vi "空载计算.vi"(10 "扭矩数组":dbl[](array[numeric])) -> (0 "空载扭差":dbl format="%#.2f", 1 "空载平均扭矩":dbl format="%#.2f", 2 "空载最小扭矩":dbl, 3 "空载峰值扭矩":dbl format="%#.2f")   [LabVIEW 2011]
panel:
  out "第一个子数组":dbl[](array[numeric])
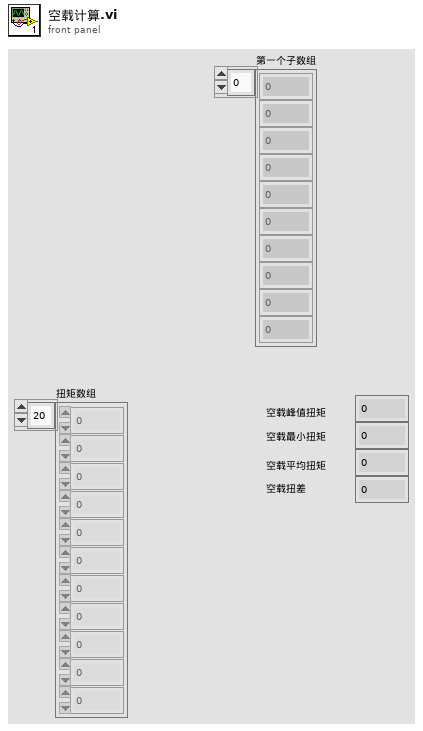
[diagram p1: front panel]
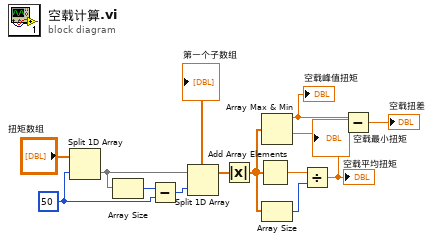
[diagram p0: block diagram]
diagram:
  w3 = 50 ("索引")
  n1 = Split 1D Array(array="扭矩数组", index=w3) -> (second subarray=w5:dbl[])  [unwired: 1 out]
  n2 = Array Size(array=w5) -> (size(s)=w4:i32)
  n3 = Subtract(x=w4, y=w3) -> (x-y=w2:i32)
  n4 = Split 1D Array(array=w5, index=w2) -> (first subarray=w9:dbl[])  [unwired: 1 out]
  "第一个子数组" <- w9
  n5 = Absolute Value(x=w9) -> (abs(x)=w11:dbl[])
  n6 = Add Array Elements(numeric array=w11) -> (sum=w12:dbl)
  n7 = Array Max & Min(array=w11) -> (max value=w8:dbl, min value=→"空载最小扭矩":dbl)  [unwired: 2 out]
  "空载峰值扭矩" <- w8
  n8 = Array Size(array=w11) -> (size(s)=w10:i32)
  n9 = Divide(x=w12, y=w10) -> (x/y=w7:dbl)
  "空载平均扭矩" <- w7
  n10 = Subtract(x=w8, y=w7) -> (x-y=→"空载扭差":dbl)
